vi "On Compile Action VI Name.vi"(11 "CD Template in":refnum<class "NIVS_Inline HW Interface (Inline-Async).lvclass">) -> (2 "On Compile Action VI Name":string)   [LabVIEW 2019, in "NIVS_Inline HW Interface (Inline-Async).lvclass"]
uses:
  NIVS_Inline HW Interface (Inline-Async).lvclass
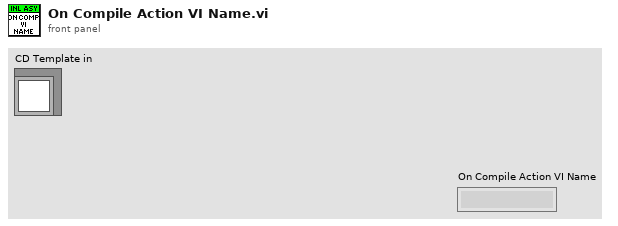
[diagram p1: front panel]
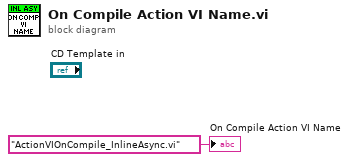
[diagram p0: block diagram]
diagram:
  "On Compile Action VI Name" <- "ActionVIOnCompile_InlineAsync.vi" ("On Compile Action VI Name")
